vi "abrir_config_adq.vi"(11 "ABRIR":bool) -> ()   [LabVIEW 2019]
uses:
  formato_aquisicao_global_adq.vi
  comunicacao.vi
  Aplicacao_atual_global_adq.vi
panel:
  in  "Array":string[](array[string])=["Deslocamento_Retirada_por_Baixo", "Deslocamento_Retirada_por_Cima"]
  in  "formato de aquisicao":bool
  in  "CONFIRMAR":bool
  in  "APLICACAO":string(combo)
  # "Selecione a Aplicacao \n       de trabalho"
  # "Selecione o formato\n       de aquisição"
  # "WIRELESS"
  # "NATIONAL"
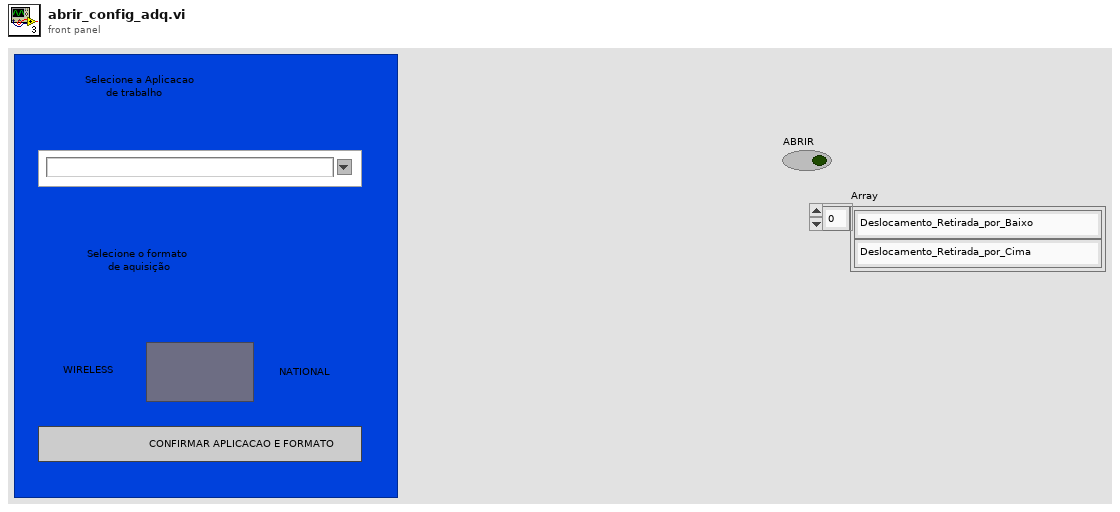
[diagram p1: front panel]
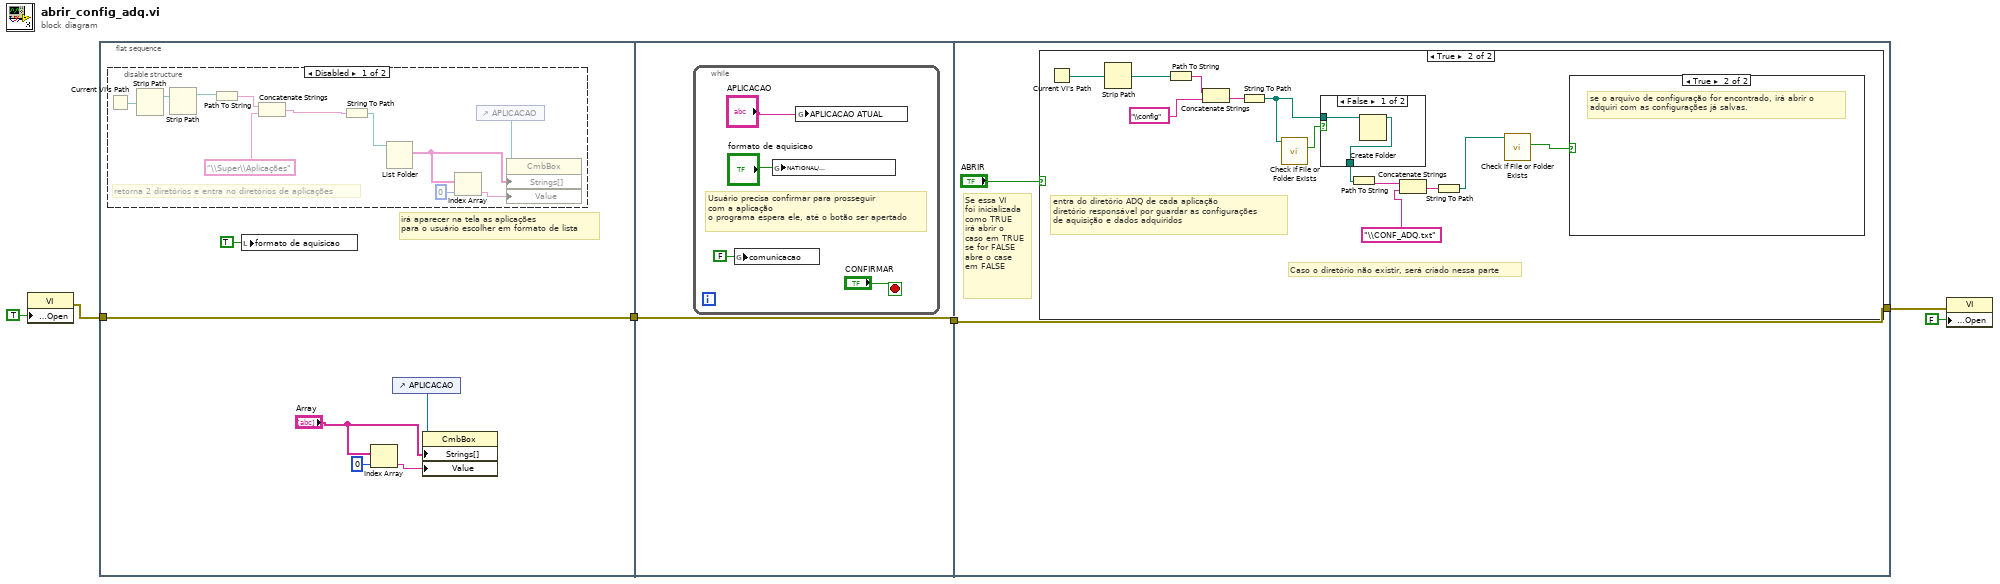
[diagram p0: block diagram]
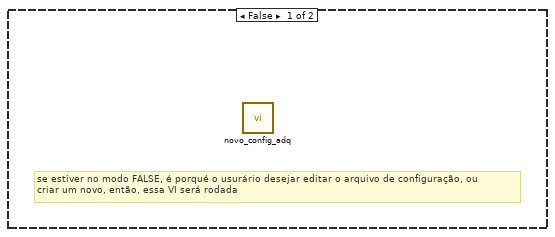
[diagram p3: hidden frame]
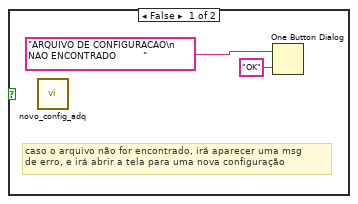
[diagram p5: hidden frame]
diagram:
  n1 = property class="VI"("Front Panel.Open"=TRUE ("Front Panel Window:Open")) -> (error out=w5:errorcluster)  [unwired: 2 in, 1 out]
  n2 = flat-sequence {
    tunnel: w5 -> [w12]
    tunnel: [w12] -> w3
    tunnel: [w24] -> w4
    tunnel: w3 -> [w24]
    tunnel: w4 -> [w30]
    tunnel: [w30] -> w1
    frame #0 {
      # "irá aparecer na tela as aplicações\npara o usuário escolher em formato de lista"
      n3 = disable-structure shown="Disabled" {
        frame Disabled {
          # "retorna 2 diretórios e entra no diretórios de aplicações"
          n4 = Current VI's Path() -> (path=w21:path)
          n5 = Strip Path(path=w21) -> (stripped path=w20:path)  [unwired: 1 out]
          n6 = Strip Path(path=w20) -> (stripped path=w19:path)  [unwired: 1 out]
          n7 = Path To String(path=w19) -> (string=w23:string)
          n8 = Concatenate Strings(w23, "\\Super\\Aplicações" ("string")) -> (w17:string)
          n9 = String To Path(string=w17) -> (path=w18:path)
          n10 = List Folder(path=w18) -> (folder names=w15:string[])  [unwired: 3 in, 3 out]
          n11 = Index Array(array=w15, index=0) -> (element=w13:string)
          n12 = control-ref of="APLICACAO"() -> (w16:refnum<vi>)
          n13 = property class="CmbBox"(reference=w16, "Strings[]"=w15, "Value"=w13) -> ()  [unwired: 1 in, 2 out]
        }
        frame Enabled {
        }
      }
      n14 = local write "formato de aquisicao"(TRUE ("formato de aquisicao")) -> ()
      n15 = Index Array(array="Array", index=0) -> (element=w10:string)
      n16 = control-ref of="APLICACAO"() -> (w8:refnum<vi>)
      n17 = property class="CmbBox"(reference=w8, "Strings[]"="Array", "Value"=w10) -> ()  [unwired: 1 in, 2 out]
    }
    frame #1 {
      n18 = while {
        stop <- "CONFIRMAR" stop-if-true
        # "Usuário precisa confirmar para prosseguir \ncom a aplicação\no programa espera ele, até o botão ser apertado"
        n19 = global write "comunicacao.vi" "comunicacao"(FALSE ("comunicacao")) -> ()
        n20 = global write "formato_aquisicao_global_adq.vi" "NATIONAL/\nWIRELESS"("formato de aquisicao") -> ()
        n21 = global write "Aplicacao_atual_global_adq.vi" "APLICACAO ATUAL"("APLICACAO") -> ()
      }
    }
    frame #2 {
      # "Se essa VI \nfoi inicializada\ncomo TRUE\nirá abrir o \ncaso em TRUE\nse for FALSE\nabre o case \nem FALSE"
      n22 = case shown="True" "ABRIR" {
        frame False {
          # "se estiver no modo FALSE, é porqué o usurário desejar editar o arquivo de configuração, ou \ncriar um novo, então, essa VI será rodada"
          n23 = call "novo_config_adq.vi"() -> ()  [unwired: 12 in]
        }
        frame True {
          # "Caso o diretório não existir, será criado nessa parte"
          # "entra do diretório ADQ de cada aplicação\ndiretório responsável por guardar as configurações \nde aquisição e dados adquiridos"
          n24 = Current VI's Path() -> (path=w42:path)
          n25 = Strip Path(path=w42) -> (stripped path=w31:path)  [unwired: 1 out]
          n26 = Path To String(path=w31) -> (string=w43:string)
          n27 = Concatenate Strings(w43, "\\config" ("string")) -> (w41:string)
          n28 = String To Path(string=w41) -> (path=w32:path)
          n29 = call <vilib>:"Check if File or Folder Exists.vi"("path"=w32) -> ("file or folder exists?"=w34:bool)  [unwired: 8 in, 2 out]
          n30 = case shown="False" w34 {
            tunnel: [w45 w46] -> w33
            tunnel: w32 -> [w44 w46]
            frame False {
              n31 = Create Folder(path (use dialog)=w44) -> (created path=w45:path)  [unwired: 2 in, 2 out]
            }
            frame True {
            }
          }
          n32 = Path To String(path=w33) -> (string=w38:string)
          n33 = Concatenate Strings(w38, "\\CONF_ADQ.txt" ("string")) -> (w36:string)
          n34 = String To Path(string=w36) -> (path=w35:path)
          n35 = call <vilib>:"Check if File or Folder Exists.vi"("path"=w35) -> ("file or folder exists?"=w39:bool)  [unwired: 8 in, 2 out]
          n36 = case shown="True" w39 {
            frame False {
              # "caso o arquivo não for encontrado, irá aparecer uma msg \nde erro, e irá abrir a tela para uma nova configuração"
              n37 = call "novo_config_adq.vi"() -> ()  [unwired: 12 in]
              n38 = One Button Dialog(message="ARQUIVO DE CONFIGURACAO\n    NAO ENCONTRADO         ", button name ("OK")="OK") -> ()  [unwired: 1 out]
            }
            frame True {
              # "se o arquivo de configuração for encontrado, irá abrir o \nadquiri com as configurações já salvas."
            }
          }
        }
      }
    }
  }
  n39 = property class="VI"(error in=w1, "Front Panel.Open"=FALSE ("Front Panel Window:Open")) -> ()  [unwired: 1 in, 2 out]
